vi "Add Pulse Recorder2.vi"(6 "Reset":bool, 8 "error in (no error)":errorcluster, 9 "Auto launch":bool=TRUE, 10 "Module type":T1, 11 "Monitor-Pulse in":refnum<class "LabActor.lvclass">) -> (0 "error out":errorcluster, 3 "Monitor-Pulse out":refnum<class "LabActor.lvclass">)   [LabVIEW 2018, in "LabActor.lvclass"]
uses:
  LabActor.lvclass
  C:/github/2018/LabActor/Controllers/Application Controller/Application Controller.lvclass
  Controllers/Application Controller/Module Types.ctl
  LabActor.lvclass/LabActor.ctl
  Controllers/Application Controller/Application Controller.lvclass/Application Controller.ctl
  Controllers/Application Controller/Read Monitor ref.vi
  NHMFL_Core/Libraries/Queued Listbox/Queued Listbox.xctl
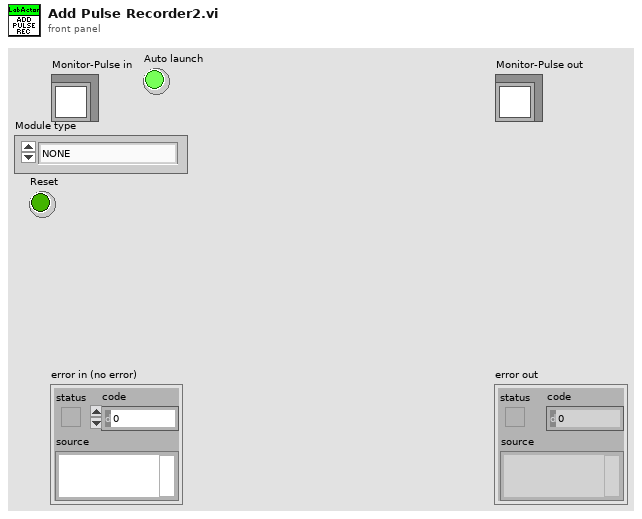
[diagram p1: front panel]
types:
  T1 = typedef "Module Types.ctl" = enum16{"NONE", "NI-DAQmx", "NI-Scope", "Red Pitaya Digitizer", "GaGe", "VISA Device", "Red Pitaya Lockin", "Monitor Controller", "Pulse Controller", "Integrate Pulse", "Lockin Processor", "File converter", "NHMFL Synthesizer", "Micron Hyperion", "Spectrum Recorder", "Resonance Detector", "TCP Communications", "Format Resonances", "Ruby Spectra", "PID Controller"}
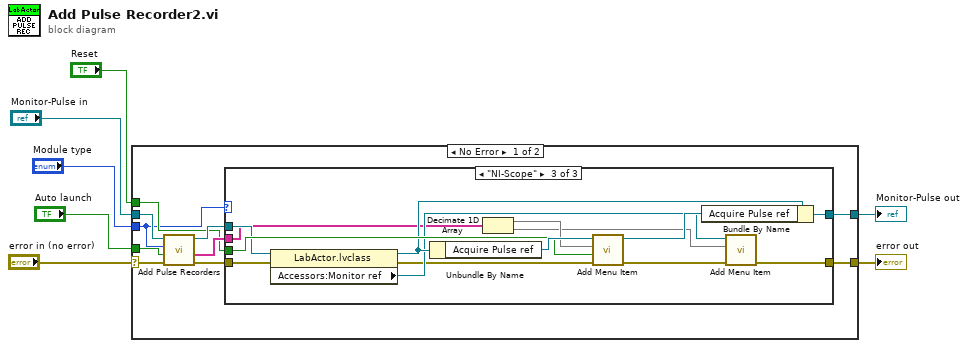
[diagram p0: block diagram]
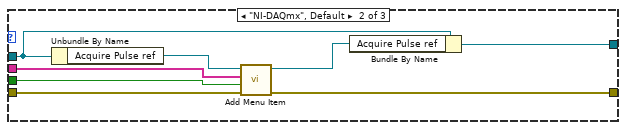
[diagram p3: hidden frame]
diagram:
  n1 = case shown="No Error" "error in (no error)" {
    selector: "error in (no error)" -> [w10 w43]
    tunnel: [w9 w43] -> w6
    tunnel: [w11 w42] -> w4
    tunnel: "Monitor-Pulse in" -> [w17 w42]
    tunnel: "Module type" -> [w8 _]
    tunnel: "Auto launch" -> [w16 _]
    tunnel: "Reset" -> [w13 _]
    frame No Error {
      n2 = call-dynamic "Add Pulse Recorders.vi"("error in (no error)"=w10, "Auto launch"=w16, "Module type"=w8, "Monitor-Pulse in"=w17) -> ("error out"=w12:errorcluster, "Actor names out"=w14:string[], "Monitor-Pulse out"=w15:refnum<class "LabActor.lvclass">)  [unwired: 3 in, 2 out]
      n3 = case shown="\"NI-Scope\"" w8 {
        tunnel: w15 -> [w19 w27 w36]
        tunnel: w14 -> [_ w25 w33]
        tunnel: w13 -> [_ w24 w40]
        tunnel: w12 -> [w18 w23 w39]
        tunnel: [w19 w22 w38] -> w11
        tunnel: [w18 w20 w28] -> w9
        frame "NONE" {
        }
        frame "NI-DAQmx", Default {
          n4 = Unbundle By Name(w27) -> ("Acquire Pulse ref"=w26:refnum<vi>)
          n5 = call "Add Menu Item.vi"("error in (no error)"=w23, "Reset"=w24, "Item Names"=w25, "Queed Listbox ref"=w26) -> ("error out"=w20:errorcluster, "Queed Listbox ref out"=w21:refnum<vi>)  [unwired: 5 in, 1 out]
          n6 = Bundle By Name(cluster=w27, "Acquire Pulse ref"=w21) -> (w22:refnum<class "LabActor.lvclass">)
        }
        frame "NI-Scope" {
          n7 = property class="LabActor.lvclass"(reference=w36, error in=w39) -> (reference out=w35:refnum<class "LabActor.lvclass">, error out=w30:errorcluster, "Accessors:Monitor ref"=w34:refnum<vi>)
          n8 = Unbundle By Name(w35) -> ("Acquire Pulse ref"=w41:refnum<vi>)
          n9 = Decimate 1D Array(w33) -> (w32:string[], w31:string[])
          n10 = call "Add Menu Item.vi"("error in (no error)"=w30, "Reset"=w40, "Item Names"=w32, "Queed Listbox ref"=w41) -> ("error out"=w29:errorcluster, "Queed Listbox ref out"=w37:refnum<vi>)  [unwired: 5 in, 1 out]
          n11 = Bundle By Name(cluster=w35, "Acquire Pulse ref"=w37) -> (w38:refnum<class "LabActor.lvclass">)
          n12 = call "Add Menu Item.vi"("error in (no error)"=w29, "Item Names"=w31, "Queed Listbox ref"=w34) -> ("error out"=w28:errorcluster)  [unwired: 6 in, 2 out]
        }
      }
    }
    frame Error {
    }
  }
  "error out" <- w6
  "Monitor-Pulse out" <- w4
